vi "add.data.to.buffer.vi"(8 "buffer.length":u8, 9 "buffer":u64[](array[numeric])=[0, 0, 0, 0, 0, 0, 0, 0, 0] format="%.0x", 10 "data":T1={"enabled"=[FALSE, FALSE, FALSE, FALSE, FALSE, FALSE, FALSE, FALSE], "byte"=[0, 0, 0, 0, 0, 0, 0, 0]} {"byte" format="%.0x"}, 11 "data.valid":bool) -> (2 "buffer.out":u64[](array[numeric]) format="%.0x", 3 "buffer.length.out":u8)   [LabVIEW 2022 SP3]
uses:
  data.ctl
panel:
  out "x rotated left by y":u64 format="%.0x"
  out "y":i8 format="%.0x"
  out "mask 2":u64 format="%.0x"
  out "mask":u64 format="%.0x"
  out "x .or. y?":u64 format="%.0x"
  out "old.value":u64 format="%.0x"
  out "new.value.u64":u64 format="%.0x"
  out "# of existing\nitems":u8
  out "Index":u8
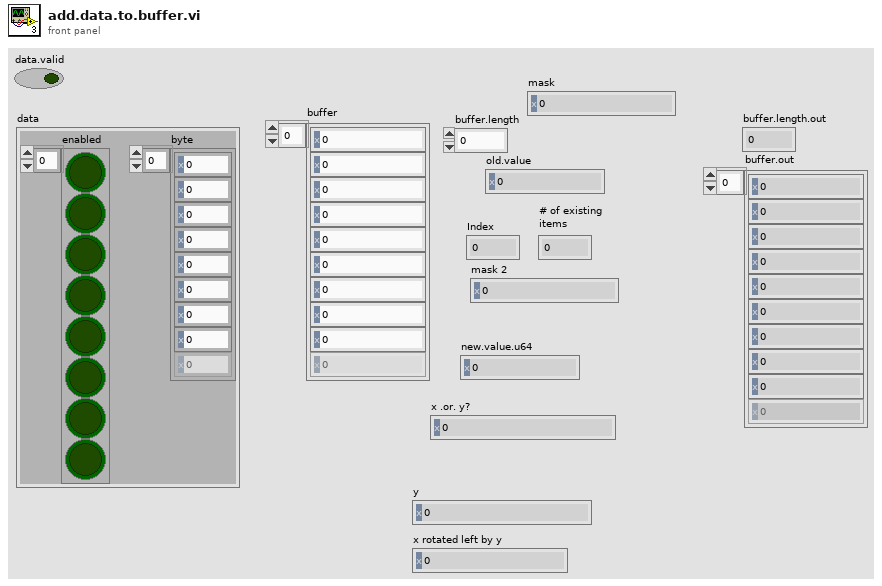
[diagram p1: front panel]
types:
  T1 = typedef "data.ctl" = cluster{"enabled":bool[], "byte":u8[]}
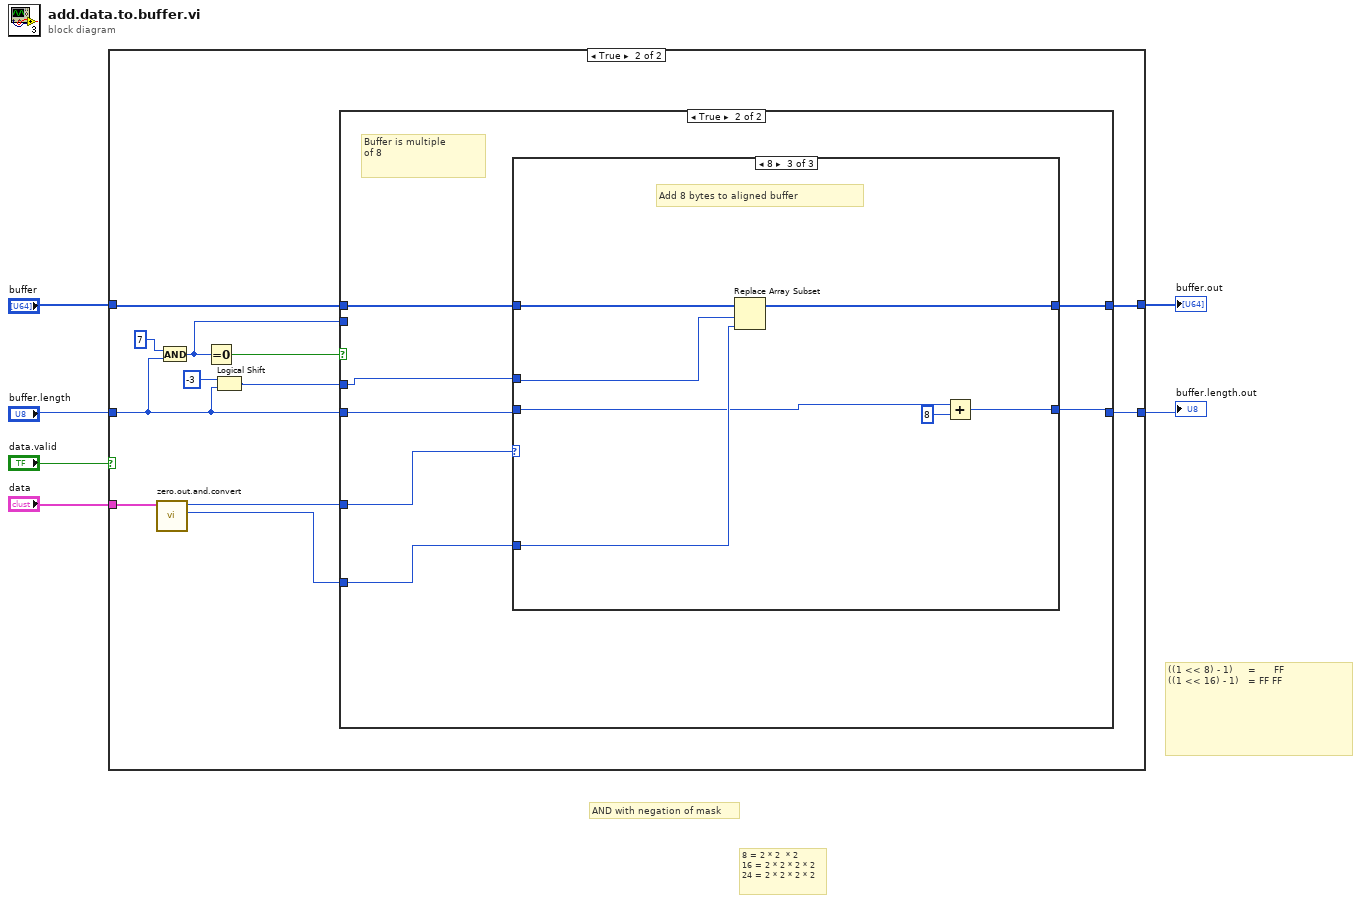
[diagram p0: block diagram]
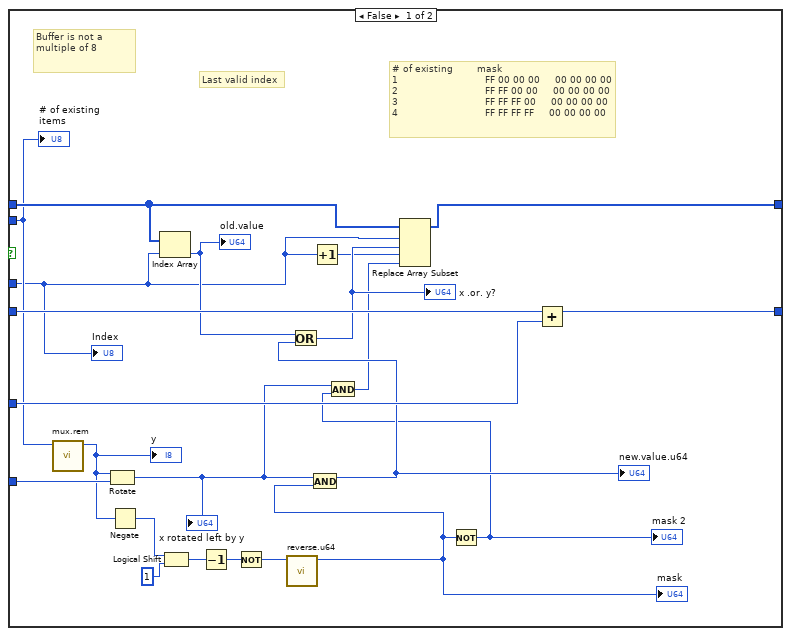
[diagram p3: hidden frame]
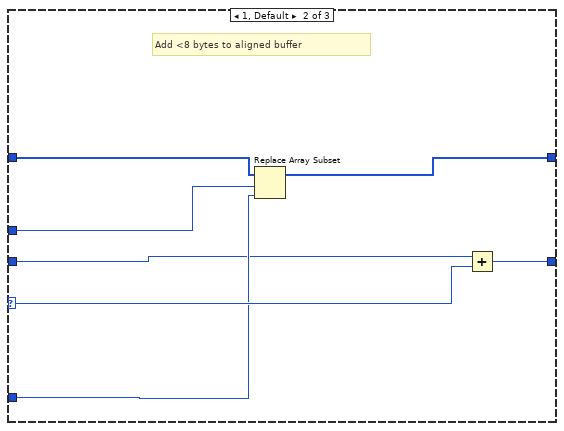
[diagram p5: hidden frame]
diagram:
  # "AND with negation of mask"
  # "8 = 2 * 2  * 2\n16 = 2 * 2 * 2 * 2\n24 = 2 * 2 * 2 * 2"
  # "((1 << 8) - 1)     =      FF\n((1 << 16) - 1)   = FF FF"
  n1 = case shown="True" "data.valid" {
    tunnel: "buffer.length" -> [w7 w15]
    tunnel: [w8 w19] -> w4
    tunnel: "buffer" -> [w8 w20]
    tunnel: [w7 w16] -> w2
    tunnel: "data" -> [_ w11]
    frame False {
      # "Data is not valid\nnoop"
    }
    frame True {
      n2 = call "zero.out.and.convert.vi"("data"=w11) -> ("u64.be"=w10:u64, "Num.of.True"=w9:u8)  [unwired: 9 in]
      n3 = And(x=u8 7, y=w15) -> (x .and. y?=w12:u8)
      n4 = Equal To 0?(x=w12) -> (x = 0?=w17:bool)
      n5 = Logical Shift(y=i16 -3, x=w15) -> (x << y=w13:u8)
      n6 = case shown="True" w17 {
        tunnel: w20 -> [w41 w49]
        tunnel: [w39 w48] -> w19
        tunnel: w10 -> [w37 w47]
        tunnel: w9 -> [w35 w46]
        tunnel: w15 -> [w42 w45]
        tunnel: [w36 w44] -> w16
        tunnel: w13 -> [w26 w43]
        tunnel: w12 -> [w34 _]
        frame False {
          # "# of existing        mask\n1                             FF 00 00 00     00 00 00 00\n2                             FF FF 00 00     00 00 00 00\n3                             FF FF FF 00     00 00 00 00\n4                             FF FF FF FF     00 00 00 00"
          # "Last valid index"
          # "Buffer is not a\nmultiple of 8"
          n7 = call "mux.rem.vi"("# of existing\nitems 3"=w34) -> ("y"=w31:i8)  [unwired: 10 in]
          "y" <- w31
          n8 = Rotate(1:w37, 2:w31) -> (0:w24:u64)
          "x rotated left by y" <- w24
          n9 = Negate(x=w31) -> (-x=w30:i8)
          n10 = Index Array(array=w41, index=w26) -> (element=w38:u64)
          "old.value" <- w38
          n11 = Logical Shift(y=w30, x=u64 1) -> (x << y=w33:u64)
          n12 = Decrement(x=w33) -> (x-1=w29:u64)
          n13 = Not(x=w29) -> (.not. x?=w28:u64)
          n14 = call "reverse.u64.vi"("U64.in"=w28) -> ("U64.reversed"=w21:u64)  [unwired: 10 in]
          "mask" <- w21
          n15 = And(x=w24, y=w21) -> (x .and. y?=w27:u64)
          "new.value.u64" <- w27
          n16 = Or(x=w38, y=w27) -> (x .or. y?=w40:u64)
          "x .or. y?" <- w40
          n17 = Increment(x=w26) -> (x+1=w25:u8)
          n18 = Not(x=w21) -> (.not. x?=w23:u64)
          "mask 2" <- w23
          n19 = And(x=w24, y=w23) -> (x .and. y?=w22:u64)
          n20 = Replace Array Subset(array=w41, new element #1=w40, index #1=w26, new element #2=w22, index #2=w25) -> (w39:u64[])
          n21 = Add(x=w42, y=w35) -> (x+y=w36:u8)
          "Index" <- w26
          "# of existing\nitems" <- w34
        }
        frame True {
          # "Buffer is multiple\nof 8"
          n22 = case shown="8" w46 {
            selector: w46 -> [_ w55 _]
            tunnel: w49 -> [w51 w58 w65]
            tunnel: w47 -> [_ w54 w64]
            tunnel: [w51 w57 w63] -> w48
            tunnel: [w50 w56 w61] -> w44
            tunnel: w45 -> [w50 w53 w62]
            tunnel: w43 -> [_ w52 w59]
            frame 0 {
              # "No new data\nnoop"
            }
            frame 1, Default {
              # "Add <8 bytes to aligned buffer"
              n23 = Replace Array Subset(array=w58, new element=w54, index=w52) -> (w57:u64[])
              n24 = Add(x=w53, y=w55) -> (x+y=w56:u8)
            }
            frame 8 {
              # "Add 8 bytes to aligned buffer"
              n25 = Replace Array Subset(array=w65, new element=w64, index=w59) -> (w63:u64[])
              n26 = Add(x=w62, y=u8 8) -> (x+y=w61:u8)
            }
          }
        }
      }
    }
  }
  "buffer.out" <- w4
  "buffer.length.out" <- w2
